vi "SandwitchingValues.vi"(8 "DesiredAngle":dbl, 10 "Angle Array":dbl[](array[numeric])) -> (3 "Angle Indexes":dbl[](array[numeric]))   [LabVIEW 2012, in "LinearInterpolation.lvclass"]
doc: "Determines indecies of angles in the input array sandwitching the desired Array"
uses:
  LinearInterpolation.lvclass
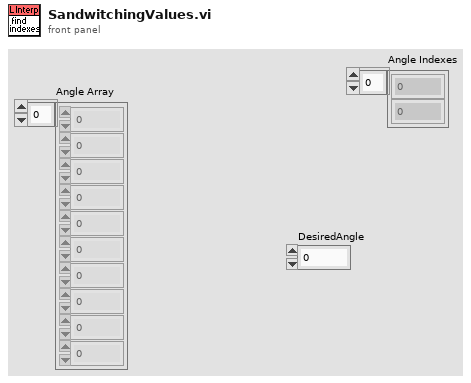
[diagram p1: front panel]
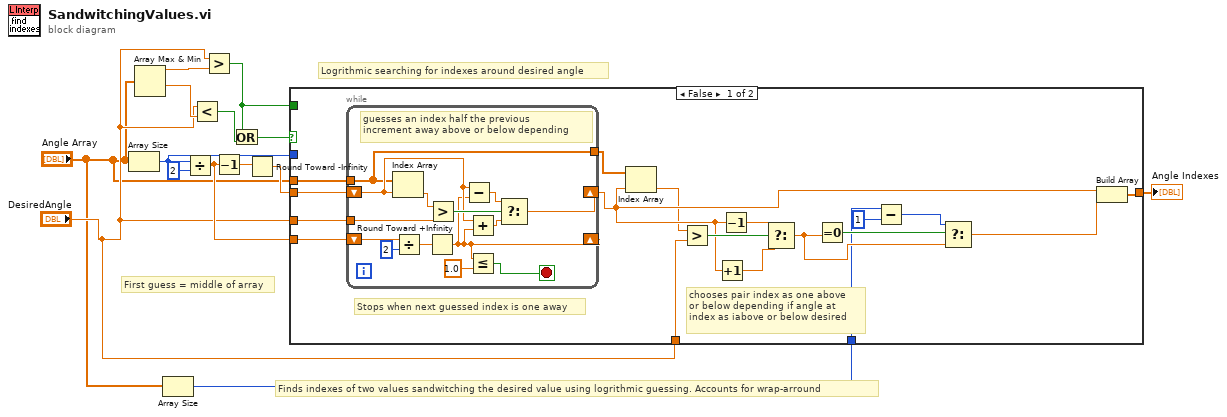
[diagram p0: block diagram]
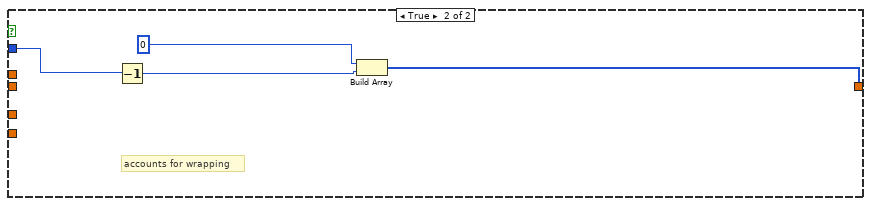
[diagram p2: hidden frame]
diagram:
  # "Logrithmic searching for indexes around desired angle"
  # "First guess = middle of array"
  # "Finds indexes of two values sandwitching the desired value using logrithmic guessing. Accounts for wrap-arround"
  n1 = Array Size(array="Angle Array") -> (size(s)=w10:i32)
  n2 = Array Max & Min(array="Angle Array") -> (max value=w6:dbl, min value=w8:dbl)  [unwired: 2 out]
  n3 = Array Size(array="Angle Array") -> (size(s)=w1:i32)
  n4 = Divide(x=w10, y=2) -> (x/y=w13:dbl)
  n5 = Less?(x="DesiredAngle", y=w8) -> (x < y?=w11:bool)
  n6 = Greater?(x="DesiredAngle", y=w6) -> (0:w7:bool)
  n7 = Decrement(x=w13) -> (x-1=w4:dbl)
  n8 = Or(x=w7, y=w11) -> (x .or. y?=w12:bool)
  n9 = Round Toward -Infinity(1:w4) -> (0:w3:dbl)
  n10 = case shown="False" w12 {
    tunnel: "Angle Array" -> [w32 _]
    tunnel: w3 -> [w31 _]
    tunnel: w13 -> [w30 _]
    tunnel: "DesiredAngle" -> [w29 _]
    tunnel: [w25 w47] -> w9
    tunnel: w7 -> [_ _]
    tunnel: w10 -> [_ w50]
    tunnel: "DesiredAngle" -> [w21 _]
    tunnel: w1 -> [w17 _]
    frame False {
      # "Stops when next guessed index is one away"
      # "chooses pair index as one above  \nor below depending if angle at \nindex as iabove or below desired"
      n11 = while {
        tunnel: w32 -> [w33]
        tunnel: w29 -> [w45]
        shift-right: [w40] -> w23
        shift-left: w31 -> [w41]
        shift-right: [w34] -> _
        shift-left: w30 -> [w37]
        tunnel: [w33] -> w24
        stop <- w35 stop-if-true
        # "guesses an index half the previous \nincrement away above or below depending"
        n12 = Index Array(array=w33, index=w41) -> (element=w46:dbl)
        n13 = Divide(x=w37, y=2) -> (x/y=w39:dbl)
        n14 = Round Toward +Infinity(x=w39) -> (ceil(x): smallest int >= x=w34:dbl)
        n15 = Greater?(x=w46, y=w45) -> (0:w44:bool)
        n16 = Subtract(x=w41, y=w34) -> (x-y=w43:dbl)
        n17 = Add(x=w41, y=w34) -> (x+y=w42:dbl)
        n18 = Less Or Equal?(x=w34, y=1.0) -> (x <= y?=w35:bool)
        n19 = Select(t=w43, s=w44, f=w42) -> (s? t:f=w40:dbl)
      }
      n20 = Index Array(array=w24, index=w23) -> (element=w22:dbl)
      n21 = Greater?(x=w22, y=w21) -> (0:w28:bool)
      n22 = Increment(x=w23) -> (x+1=w26:dbl)
      n23 = Decrement(x=w23) -> (x-1=w27:dbl)
      n24 = Select(t=w27, s=w28, f=w26) -> (s? t:f=w19:dbl)
      n25 = Equal To 0?(x=w19) -> (x = 0?=w20:bool)
      n26 = Subtract(x=w17, y=1) -> (x-y=w15:i32)
      n27 = Select(t=w15, s=w20, f=w19) -> (s? t:f=w18:dbl)
      n28 = Build Array(w23, w18) -> (w25:dbl[])
    }
    frame True {
      # "accounts for wrapping"
      n29 = Decrement(x=w50) -> (x-1=w48:i32)
      n30 = Build Array(0 ("t"), w48) -> (w47:i32[])
    }
  }
  "Angle Indexes" <- w9
